vi "UHR-Fleezers Control (host) -Leonardo 04-2018 V2.vi"(0 "Tab Control":T5(tab)=enum."Trap Control (RF)") -> ()   [LabVIEW 2013] (continued)
-109.41462449554598, -109.30248158488335, -108.70735295493108, -109.9174743694956, -109.94232543385962, -110.71725446170196, -110.0346196158573, -110.34814317845934, -110.6651078322521, -107.55409880424479, -108.71734776861287, -109.50902203986271, -110.40207542979611, -108.7847687630861, -111.10599488129682, -109.30824728923263, -108.20134064331717, -110.55959112431609, -107.77099734327174, -110.23862843385446, -108.48520797666865, -108.54205896654946, -107.79288769037599, -109.84022250170581, -108.02758364115576, -109.35132492327935, -108.87009749667932, -109.86905123364855, -109.19826752168308, -106.835240323691, -109.37910022114056, -110.80633973102931, -109.12703823829597, -111.07432699570984, -111.8064506085314, -110.09349947650527, -108.66467295777367, -108.75119108236053, -112.63983351316729, -110.90940743670113, -110.27973159222081, -109.57141664526549, -108.61645363771719, -109.31742355616147, -109.5839599160637, -110.01188998365383, -110.01923429741011, -108.94779759137936, -108.26169431000017, -109.24553201026085, -109.95709526422822, -110.68677343596859, -108.7678734483002, -110.47090469179284, -110.31604700116512, -110.10256600741997, -109.76634647265719, -110.8830805828562, -109.94609564072982, -109.20662382740542, -108.12492970530919, -110.5274435478767, -108.02351960398035, -110.6264936805739, -107.14559226383577, -109.13821777857531, -111.05324489472586, -110.15190797512811, -107.96366234783144, -110.03950681967147, -109.17476300510336, -110.41251816187909, -111.39219865477246, -111.32530426869943, -109.97369363558423, -108.98666403063845, -109.62049358645565, -109.58130494498671, -111.72738873188874, -110.39825891106616, -108.57430325757545, -111.28625510212446, -108.77421250595326, -109.75025415031793, -109.51948456745635, -108.82129398637998, -109.81362137198361, -107.86292494316123, -107.49318292857053, -109.66948564589373, -109.54288390056654, -107.99912445612077, -110.3497559614379, -108.00549349666127, -110.01361420523357, -108.4977916421456, -109.67078387286976, -109.85678367732866, -112.01237658746248, -108.4855625950998, -110.84880875737286, -110.9178674382154, -110.44187536727453, -108.75076921971127, -110.04946286646651, -109.99780941000827, -110.14242932305507, -109.56343773672316, -109.6278993388131, -108.77419573790174, -109.10543670530926, -109.7801848627463, -110.30733124104881, -113.13440550301436, -109.32709134514755, -109.74136656933283, -110.01525283266193, -109.43924662938396, -110.25325289253, -107.75460576671303, -110.60057027395933, -110.71458404922404, -110.15788509050662, -110.69167485018224, -110.96006652476157, -111.01156633983031, -111.6058448010008, -109.51364005052672, -109.76058205940885, -108.43421621088261, -109.47973949170208, -109.25533250208288, -109.47422603921065, -111.36411644613841, -107.27566171102698, -110.45098686173688, -109.93589296291184, -109.03803734663714, -110.53118128434016, -110.2408872254969, -110.0532234862915, -109.94185495614619, -110.2662004220774, -109.51094016962288, -108.5210104215432, -108.13691752270934, -110.18460088390265, -108.32609309150783, -109.89652230508281, -109.80923900768477, -109.01917388968883, -110.01248300968739, -109.43415605440147, -108.09823485138017, -107.40637725320931, -109.40632232658412, -111.97981999127656, -111.16609811629485, -111.64500793960192, -110.99793748693381, -109.55531276386903, -110.2535662621666, -108.17429802469516, -109.09425673355422, -110.23187110421917, -110.55358397926925, -109.93461124753053, -109.55604345832225, -109.44569510408274, -109.72185151080762, -109.52963702944834, -109.2303630328152, -109.74819502244243, -109.3932530349457, -109.17096788339686, -110.46153727064616, -113.1073731246639, -109.43753070459397, -108.13332547768168, -109.42294574929969, -108.45798401969856, -110.29453435046327, -112.66249403705643, -108.78314667434937, -105.9634478773668, -109.14327524669528, -108.50645190860273, -100.81571594994128, -104.4482859840643, -110.68926237051092, -109.12362553230196, -109.45234390564677, -107.91461416156068, -110.67788819353727, -110.05744935668449, -111.78333392154664, -106.83628914455993, -110.11115457346548, -109.13434608275826, -110.80006861194663, -110.35323502651462, -112.29149906501372, -109.01656376530778, -109.30871662948859, -109.79736315392456, -109.17848983603582, -108.09752397056482, -111.6039030763455, -109.27008844877828, -110.84475733314184, -109.72393917557073, -111.31060762894991, -110.78858793807466, -107.12841545099752, -109.54510865218204, -105.2805426080281, -106.28514149354733, -109.50656759582803, -110.14700878401054, -110.49737016725709, -109.19811547071924, -109.92527399676051, -110.7961615015146, -109.7447227818197, -109.49432012009893, -108.714081576733, -110.09766801550917, -109.08448507943001, -110.36154838733857, -109.86328656267403, -109.21144237434696, -112.4145136888034, -108.57567151011159, -109.66748589540896, -109.72985837578446, -109.29989238126763, -109.85868902806475, -111.01778182304162, -111.23625326328558, -110.01270868104203, -109.27067928081415, -109.71171312410247, -109.28697459293629, -110.67868067201007, -110.91353786857455, -111.21479955051575, -109.11315965407708, -109.40418681804496, -107.80511819596003, -107.37201025889816, -111.81969609169838, -109.89875624306032, -110.29328043898657, -109.74853280072202, -111.39527865400605, -109.47746221101964, -111.75141177452517, -109.31325306583483, -109.30117448911659, -109.3997781364162, -109.45356931295724, -109.60585285774386, -111.33951689512735, -107.74187210470228, -109.62706021606415, -108.72139655505221, -109.79552836110567, -110.64354037499807, -110.96138240913136, -110.02215059889615, -110.92978442698893, -110.0620778287114, -110.85019647293322, -111.77397403227091, -109.81257196800128, -109.15643451383403, -110.72777566469594, -108.7463769025616, -109.80959395914073, -111.24500986151126, -110.48863498350322, -110.30863780110901, -109.79331354195703, -110.34087081762074, -109.45183222569266, -109.6440990067103, -111.15034876658994, -112.14912485578341, -111.8886180186196, -110.57054820211916, -111.07556239924551, -110.5872832735073, -110.28912501038172, -108.91501133754849, -111.44575118962761, -109.90799859177967, -109.74421995550023, -108.70941446115883, -110.28822893097275, -109.70039554000401, -110.33701797570251, -110.79445894683306, -109.57694314608153, -108.816904416038, -109.66517126767175, -109.39501469321644, -110.85775022889956, -109.3689402795614, -112.09107318723095, -110.67985626248422, -110.32971146814747, -112.08166943494875, -109.93955548712543, -109.31722953035252, -110.2062913031861, -108.22565380081006, -110.680898028151, -111.95386604441454, -110.83354130587097, -108.5873626748948, -111.97536144124408, -109.23944159551515, -111.57859477689586, -110.80135186615524, -110.4800953731021, -110.14040729648133, -109.25873050390551, -108.87000960474569, -110.97091597211167, -110.15787270199012, -111.62434537618091, -108.5421625277294, -110.42258666403919, -110.96896115868603, -108.98253068925274, -109.54245055160168, -110.28051096122468, -109.48060498658319, -109.77618362117276, -111.64513838754992, -111.13945484239875, -110.18094280356001, -110.43757222770748, -110.81588360154201, -110.11656805555333, -108.47936291282355, -109.16476249859961, -109.3549985917136, -110.77753190334253, -111.46065694661178, -110.40387985996301, -109.95673803226478, -111.58660981285446, -108.59894875229345, -109.37333363882607, -110.26849699991793, -109.30500469266264, -109.23789020998296, -110.82000706486865, -109.25927538839868, -111.03285659417519, -111.08899832832414, -110.69361682858042, -109.45187168573815, -109.9614018482838, -109.70209527974106, -112.11903952100165, -109.59713611623246, -110.70292028698111, -110.12743849746808, -110.63315585514292, -108.60450276298175, -109.32832664986026, -109.99753023477764, -109.46644696130294, -109.1781290160558, -111.58830180575129, -111.67229040267557, -111.3750024136205, -108.33616679452298, -109.99797067800029, -110.50892429124391, -108.66074740829372, -111.17094662568759, -109.87538933985836, -109.152526628291, -110.44623159817101, -110.21603106403009, -110.64376935639365, -109.36897426842583, -108.67303022227141, -109.89327693080823, -111.50442955563923, -111.37532237834381, -109.38132821290205, -109.73509680539144, -110.53918379735906, -111.22869870340647, -109.39977573957616, -110.3674665334106, -110.5366125953241, -109.99025356764304, -109.97300035646616, -109.87631077033762, -109.64608829594286, -113.02486102973394, -108.26250283140733, -109.62234918138763, -111.18766216512655, -110.33666026406992, -110.5808115327039, -108.2971671321189, -110.10964334161903, -110.61254021379767, -109.89852549557533, -110.16562049054073, -109.41433790018287, -111.2453823439446, -110.45554802599901, -113.11454453784393, -110.7333866145056, -110.00858191882439, -108.54745315874294, -110.08430415376903, -111.9006972727596, -110.3031506154679, -110.26331790366497, -109.36797925566673, -109.04860552478912, -111.83514212681175, -111.38960737633833, -109.01429665187288, -110.96404839103826, -108.95488871107163, -109.09652004914592, -111.884304581971, -110.57566691021339, -111.95113404442795, -110.13677174050159, -108.10078686353354, -107.69442565416006, -112.42676605669463, -109.12681161784135, -109.23120766087519, -110.57649395555585, -110.22143082743162, -108.40065951773644, -109.46923168308618, -111.39095086729745, -110.46375658526013, -111.45145283328486, -112.22610823637353, -110.61090190564383, -112.22250292674809, -111.7379343196361, -110.18530386733481, -108.93867365671692, -111.89304844956082, -109.06146134986984, -110.98405731832798, -109.76366821333497, -108.08326795663608, -109.95041147835065, -112.94140614324155, -111.79814935135965, -108.07337559063119, -109.13733403265212, -111.74906646037496, -111.12228668433455, -110.02899450462209, -110.22237716929811, -109.0224776891049, -110.18135850497721, -113.32516073881047, -111.3576490243877, -110.60510094465171, -109.6935518470342, -110.36313473154901, -111.95933240129618, -109.49625308071019, -109.18827910216122, -110.54311407822692, -108.4811035913567, -112.81280225723607, -108.86530665787413, -110.85796435061886, -110.40059714639627, -108.19250716343407, -108.96956521802292, -108.61281798886506, -109.78061525370413, -111.58885511891798, -109.06279169160345, -111.43043988466789, -111.63169336321079, -109.54702536206447, -109.62860636296405, -109.47865811135546, -108.02265793654806, -109.97461304995515, -110.72549884050886, -111.57309413919933, -110.03317891949746, -110.39570411598524, -110.27606115470397, -110.63294457306095, -110.71821689302902, -110.38076268941819, -111.51223508887897, -110.40703572670697, -112.24933273737743, -109.74954300082398, -108.46020292937696, -111.05315219575881, -110.38635148390118, -109.58268303790976, -112.34211536832117, -108.45894118755307, -108.96463982695337, -110.56040438523046, -110.67803313671729, -111.07349872375121, -110.42184162876096, -111.82081126435692, -108.85923651136297, -112.57723799596502, -113.65690874668172, -112.62314325834605, -110.70357529341362, -110.959925221544, -111.26336183001875, -108.1350700630152, -107.94545932312926, -111.17610778209841, -110.20386728310686, -108.55646511121591, -109.8400922569145, -111.73466587035968, -110.47272877573613, -108.33011124048193, -107.93042857580332, -108.60928277989103, -109.25240966798974, -108.96403833602028, -106.94222615757475, -109.37086694261907, -106.72743097285155, -109.03160193412796, -107.3549903889451, -106.8543848510082, -107.83503929060929, -106.30745467433752, -108.36915807168845, -107.13065938379303, -107.84769200880969, -106.08004345082777, -108.15244601930225, -108.37254117816573, -106.57863034819223, -108.1283698227614, -108.19776505569902, -107.58283412238643, -108.17365133196301, -108.6794309781181, -107.91552140588759, -111.60122989270022, -107.04360635941174, -111.55535949001795, -109.39870426166594, -109.55937904851662, -111.81389508925734, -109.88957041098786, -110.84764586896561, -110.59130246272693, -111.15944135223884, -110.19496154041607, -111.51861903129362, -110.74798816525838, -111.37312965175558, -110.10842817220238, -110.73198099204856, -111.36708667993291, -110.30840247819665, -110.11744489669044, -110.55237850846444, -108.2073528237766, -112.70750856801911, -110.99917956040802, -109.84949484779976, -111.3403161887679, -110.08924435263565, -110.17749213365616, -112.10849123224503, -110.94270741299202, -109.29350963424746, -110.33477486966507, -112.19620157705627, -111.45484078395934, -111.86858843505124, -110.22491147345858, -108.96177661263177, -108.67862820579893, -107.55155410582937, -108.27984439169573, -108.72682528077233, -110.64231212183269, -109.32873093119183, -112.98564364754564, -110.78933114228725, -108.50921025910479, -107.91087245586935, -112.57350030929283, -111.75871577457525, -108.42095298945462, -112.31266064114303, -110.1295657579673, -109.67444664474456, -110.33749884929306, -109.16098218724147, -109.63554874360221, -109.15892392675141, -111.90580809179818, -108.81196712336858, -111.42223552606656, -109.90571484965518, -109.99739812086352, -111.64103850263211, -111.31463957090885, -110.61247447444549, -110.20960333715526, -110.1707327818923, -109.70412636554525, -110.97278093107532, -110.24386747740314, -109.81378546061525, -110.83784085086458, -109.77357954318757, -111.22663832948885, -111.14563050139252, -110.87152231402447, -110.34246044319893, -109.97174570657546, -110.23599592972218, -111.08206161770731, -110.0073315341242, -111.11748366902188, -112.04005964728601, -109.81290191679287, -109.68543639040858, -112.01143296194752, -110.13641850530031, -108.19348942447623, -109.7534468948808, -109.36697824644176, -97.56454580435337, -104.97829040517887, -108.1539132982256, -110.048991273122, -107.46172505860011, -110.49269280640675, -109.94209901400029, -109.38576869679022, -111.43699124347364, -110.89973083498887, -111.2994445418276, -109.25144782032437, -113.25676258473536, -110.82078737428088, -109.97779571182073, -113.36294799183014, -111.38584551238931, -112.17267897274873, -108.56430946159155, -112.06841286528645, -110.36822473102735, -109.54758527532016, -110.48190506674653, -110.03535695860182, -109.3951469796576, -112.41910682256774, -111.38124138857238, -109.37850389100952, -111.65544568836181, -111.55876881606889, -109.3029209617236, -109.20030046194076, -108.82610577621037, -110.53329453526098, -109.96090595542142, -109.67834229432077, -110.62303603007352, -109.8388817181171, -109.22430039793213, -108.92749786663613, -110.05794249283548, -109.58534943218437, -110.50493887507297, -109.96373022997366, -111.0645036323456, -111.28501675364454, -109.77386932343008, -108.8952247140968, -110.09242801628717, -112.90943444063141, -110.72299296247249, -109.39094335967056, -110.95165384057718, -109.59809519359453, -110.4978602309597, -109.67109981692639, -111.2489619905986, -110.0937750887109, -109.76771021128954, -108.32976315018955, -111.3058145792439, -111.09464974601362, -110.99797900696136, -109.174315000222, -109.630351559617, -110.26289147175856, -110.22688407202517, -109.96748050100612, -112.13247633583758, -110.59994952890855, -110.93023020153811, -109.22457750926695, -110.26162558926984, -110.09713110375579, -111.73858994918328, -109.78183160058515, -109.7603471824367, -110.96016892586911, -111.23309626937036, -109.83093663960678, -114.05354944347246, -111.58202863059464, -110.42281828744524, -110.9521484732059, -112.5120328206343, -111.614891937737, -109.84428787405484, -111.61119567831453, -110.43095563229411, -111.71833448430398, -110.01132196809407, -109.37558169247951, -109.14091380022785, -110.42663661754088, -110.3598013572826, -109.78207135281417, -109.94058843992468, -109.88210328447205, -108.6217811850147, -107.17834387173707, -110.6447226986756, -111.10704778101115, -111.24396771977769, -110.47849395539598, -110.75150631628034, -109.67662689396347, -109.23145032835053, -108.83780193265358, -109.43468321661163, -102.22521103859944, -106.90009867479111, -108.91580608784525, -109.58671397003187, -110.56692028436989, -108.75103142680105, -111.00795573084157, -110.75039085328763, -109.48222099288613, -111.8621134816908, -110.26507966786443, -108.885924716389, -109.30841399453053, -112.3188631425597, -111.05677697153163, -108.8268571902449, -109.63028152237679, -114.82339015806369, -107.03435216376964, -111.34847692589166, -109.61354114874855, -112.32687758049907, -109.59816404231358, -111.64248480241805, -111.84075757907273, -110.44017657636552, -110.15181635726277, -111.93813663582833, -109.11826378836209, -109.99779889778326, -109.927119030584, -109.4389650887841, -111.52448814187727, -111.38736268499642, -110.51920914917922, -108.64230614681055, -108.90307263595304, -110.57246891832371, -109.65575340646116, -109.80359672370373, -108.83368585528197, -111.09385004343437, -108.83430005497769, -112.37784208819113, -109.50005381621696, -109.67421750136593, -111.39664088797532, -109.70867599669316, -109.52498993629875, -111.12341349673187, -110.0484037026941, -109.55138667646308, -111.06614422098669, -109.4785941493091, -110.25724082617013, -110.93950616855716, -110.53487953881397, -111.45722057988401, -110.32393446412904, -110.34361936710438, -108.6610336097813, -109.53631603696368, -108.06930707969195, -107.68056561368934, -108.73860971027449, -108.87111384617579, -108.40433837098611, -110.55999576884835, -106.83832061167207, -108.28786975902513, -109.18482905697472, -107.81071696594883, -107.91047268802457, -108.79613111673706, -111.05361322310213, -109.97897453479862, -109.12920563729425, -111.20538391490288, -109.26286135293664, -111.31400407177502, -109.92167984752287, -110.70854322826071, -108.59406515713611, -109.69371333227458, -109.36664873267313, -110.35521729513704, -110.40667924006368, -112.0181844636846, -111.01529188207431, -110.59246505728431, -109.95068312717868, -110.75807466894047, -109.58596443762707, -111.12127793384956, -109.59041634463125, -111.56255571372793, -110.43405578864342, -108.39660324329928, -111.1420710307505, -113.64788483868595, -111.67645688353934, -111.36878760365944, -109.68523694561108, -110.11608766310304, -109.25670490330123, -110.73546181099229, -111.77855039399805, -107.9662794718261, -109.67483334602832, -109.891258579519, -110.24757768183042, -109.50202895993814, -110.07763831916637, -109.96891925839451, -110.97268925927641, -109.31698133827767, -112.27933593506792, -110.36206721075725, -109.47379463718867, -110.27836850941338, -110.63738280998388, -111.3611682777485, -110.72689155959884, -111.55480904927032, -111.16689658479412, -110.35555645743601, -111.56609319131051, -110.88279459952174, -114.73607246523177, -109.95813757295693, -107.64639932425493, -111.26486783320321, -112.03946356928121, -111.8915972448334, -110.35245920812773, -110.83155104803564, -110.67437747473863, -110.9959682920065, -110.7815352345103, -111.13722283763049, -112.54797265493127, -110.06894780898469, -111.65186554925783, -111.83545188116254, -110.65894756123697, -108.48458025065264, -112.43760714427981, -114.1368408201927, -110.40065777895025, -110.1066998945526, -108.60654239598591, -110.5716060205154, -110.74257357180736, -111.1136089342442, -111.53539811075092, -113.2559601458872, -109.2003227548348, -110.42285840441025, -111.4086884998834, -111.61503050693868, -110.8194303494779, -108.9701587059964, -112.58521089509063, -110.10873915265242, -112.43440038319561, -110.03468788439882, -111.57896603236308, -110.21939233582523, -109.03614470500777, -110.11738923539659, -109.55359574898291, -110.416473622654, -109.4626868574157, -111.17164025076731, -110.3579689035081, -109.04338716157822, -112.36157114517567, -109.32125615922843, -112.71105693789394, -110.11019129547768, -108.96439402555632, -111.107663418839, -111.48306369859839, -110.9317530461794, -107.98628540532181, -111.1636972328743, -110.47837837583148, -109.04649309175733, -110.27110334963734, -111.35803630614352, -110.77259078859605, -111.46352820533895, -111.16789261049541, -109.2376344776325, -111.6795794983659, -111.74292205167644, -109.40835022991612, -111.02163652600731, -108.79482078001607, -110.6718658416566, -111.08747067599332, -112.15383726791498, -109.47049126158717, -109.061574046483, -111.23993049318979, -111.02521156588335, -109.46012868444186, -110.13918914826291, -112.08180381836377, -110.61929875223015, -111.4424805369965, -111.43420275069585, -109.71347556238717, -110.24726273025648, -109.7860268673935, -109.94126895018422, -111.41948668868926, -108.90555991781676, -110.81242861886172, -109.65007052722677, -112.12672329335953, -110.01123170946096, -111.13980448279096, -113.92013682657084, -108.6000853867411, -110.66793592761913, -110.61237681642844, -110.00839105230496, -109.38083187034974, -109.46119372195675, -110.3708067287448, -108.55518656223285, -113.33935987443276, -111.92184778392033, -111.80820718236087, -107.36852757311246, -109.51077803361602, -110.066791721019, -108.756710558672, -107.91391289865918, -110.72851430959301, -111.39074956442978, -112.928843679455, -109.87348280521556, -112.21371750380071, -110.82495902297394, -109.94006136010094, -110.58757785050143, -110.2790091349881, -111.43884888223081, -108.09540986530712, -109.63783244641691, -110.19577975613292, -110.01690033746098, -112.75938920157155, -109.27158857362184, -111.19519821680541, -110.14381902425255, -110.45955291199236, -111.55660330002316, -110.75604254261134, -111.02122553784838, -111.6490091060193, -110.93362819419399, -110.49033159684308, -110.70789549836027, -110.41991882034145, -110.0264093421208, -109.18432746063652, -110.15292268755287, -112.40733942236504, -111.32869665965416, -110.95418667871114, -111.14291568823575, -111.75555369152653, -112.98146297069803, -109.73870744292117, -111.33806139459435, -110.18838799491355, -112.60408243005732, -110.26112648646833, -110.58257045107274, -109.75155437454112]}, ...(2 in all)]
  in  "FFT 1 Choice 1":u16(ring) items=["T1 Y", "T1 X", "T1 Sum", "T2 Y", "T2 X", "T2 Sum", "T1 FB X", "T1 FB Sum", "T2 FB X", "T2 FB Sum", "PSD Y", "PSD X", "PSD Y Sum", "none"]
  in  "FFT 2 Choice 1":u16(ring)=3 items=["T1 Y", "T1 X", "T1 Sum", "T2 Y", "T2 X", "T2 Sum", "T1 FB X", "T1 FB Sum", "T2 FB X", "T2 FB Sum", "PSD Y", "PSD X", "PSD Y Sum", "none"]
  in  "FFT 1 Choice 2":u16(ring)=1 items=["T1 Y", "T1 X", "T1 Sum", "T2 Y", "T2 X", "T2 Sum", "T1 FB X", "T1 FB Sum", "T2 FB X", "T2 FB Sum", "PSD Y", "PSD X", "PSD Y Sum", "none"]
  in  "FFT 2 Choice 2":u16(ring)=4 items=["T1 Y", "T1 X", "T1 Sum", "T2 Y", "T2 X", "T2 Sum", "T1 FB X", "T1 FB Sum", "T2 FB X", "T2 FB Sum", "PSD Y", "PSD X", "PSD Y Sum", "none"]
  in  "Compute FFT":bool
  in  "Reset FFT":bool
  in  "# Spectra to Ave.":dbl=25.0
  out "Ave. Time (s)":dbl=1.5
  out "1 Channel":waveform(dbl)(graph)={"t0"=timestamp(0 s since 1904-01-01), "dt"=1.4999999999999999e-05, "Y"=array[20000 elements], "attributes"=variant("NI_ChannelName"=variant(string "T1 Y"))}
  out "Slow mean":dbl=-0.021350993491001932 format="%0.2f"
  in  "Slow mean N ave.":dbl=1.0 min=1.0 step=1.0
  out "Mean Intensity":dbl=-0.021350993491001957
  out "Sigma":dbl=0.006231607115497778
  out "Sigma/Mean":dbl=-0.2918649719098079
  in  "Subtract mean":bool
  in  "High Res. Display":u16(ring) items=["T1 Y", "T1 X", "T1 Sum", "T2 Y", "T2 X", "T2 Sum", "T1 FB X", "T1 FB Sum", "T2 FB X", "T2 FB Sum", "PSD Y", "PSD X", "PSD Y Sum"]
  out "APD 1 Rate (Hz)":dbl format="%#_3p"
  out "Feedback overload":bool
  in  "T2 for asymmetric\n(MHz)":dbl=85.0
  in  "Middle freq for \nsymmetric (MHz)":dbl=78.0
  in  "Symmetric manual \ntrap motion":bool
  out "Stage Moving":bool
  in  "Read Cal":bool
  in  "Confocal Linescan":bool
  in  "Speed (nm/s)":dbl=100.0
  in  "Furthest Withdraw (MHz)":dbl=15.0
  in  "Confocal Image":bool
  in  "Round T1 X":bool caption="Round"
  in  "T1 offset_x (mV)":dbl=44.132512662199076 format="%#_2g"
  in  "T1 kappa_x (pN/nm)":dbl=0.1608167093260824 min=0.0 step=0.001 format="%#_2g"
  out "Time (s)":dbl=40.5
  out "Total Time (s)":dbl=60.0
  in  "Start Saving":bool
  in  "Cal sets to save":u32=50 min=1 step=1
  in  "Comment (data description)":string="testing confocal setup"
  out "Calibrating Trap...":bool
  in  "Trap 2 (ON/OFF)":bool=TRUE
  in  "Trap 1 (ON/OFF)":bool=TRUE
  in  "Save Calibration":bool
  in  "N sets to save":u32=200 caption="N Sets"
  in  "Save N Sets":bool
  out "Save file name":path=path "I:/Data/160525/160525_043.dat"
  in  "Save ave N":dbl=500.0 caption="Averaging Factor"
  out "Saving...":bool
  in  "Stop Saving":bool
  out "Progress":u16(slide) scale=0.0..100.0
  out "Manipulating Trap":bool
  out "Buffer Status":dbl(slide) scale=0.0..1.0
  out "Overflow (data lost)":bool
  in  "Reset":bool
  out "Data Rate (Hz)":dbl=66666.66666666667 caption="Trap Data Rate (Hz)" format="%#_3p"
  out "Data Period (s)":dbl=1.4999999999999999e-05 caption="Trap Data Period (s)" format="%#_6p"
  out "Save Data Rate (Hz)":dbl=133.33333333333334 caption="Rate (Hz)" format="%#_6p"
  out "Save Data Period (s)":dbl=0.0075 caption="Period (s)" format="%#_6p"
  in  "T1 alpha_x (nm/V)":dbl=701.8425766517444 step=10.0 format="%#_3g"
  in  "T2 alpha_x (nm/V)":dbl=806.869454518421 step=10.0 format="%#_3g"
  in  "T2 kappa_x (pN/nm)":dbl=0.13871102209446912 min=0.0 step=0.001 format="%#_2g"
  in  "T2 offset_x (mV)":dbl=-16.403354316809207 format="%#_2g"
  in  "BD 1 Frequency 2 (MHz)":dbl=90.0 caption="T2 X (MHz)" min=60.0 max=90.0 step=1.0 format="%#_6p"
  in  "Green Laser ON/Interlacing":bool
  in  "Round T2 X":bool caption="Round"
  in  "AO1":dbl(slide) caption="Confocal Y (V)" min=0.0 max=10.0 step=0.01 scale=0.0..10.0 scale format="%_1f"
  in  "AO2":dbl(slide) caption="Confocal X (V)" min=0.0 max=10.0 step=0.01 scale=0.0..10.0 scale format="%_1f"
  in  "Trap Raster Scan":bool
  out "Raster Scanning...":bool
  in  "Trap Delta (MHz)":dbl=20.0 step=1.0
  in  "Trap Intensity\nSetpoints (V)":cluster{"Set 1":dbl, "Set 2":dbl}={"Set 1"=3.0921353801080356, "Set 2"=2.9123813592944123}
  in  "Index":dbl=43.0 caption="Save File Index" min=1.0 step=1.0
  in  "BD 1 Frequency 1 (MHz)":dbl=70.0 caption="T1 X (MHz)" min=60.0 max=90.0 step=1.0 format="%#_6p"
  in  "Goto Top (F6)":bool
  in  "Save":bool
  in  "Capture":bool
  out "?":cluster{"x":string, "y":string, "z":string}={"x"="N.D.\r\n", "y"="N.D.\r\n", "z"="N.D.\r\n"}
  in  "Capture Locations":i32(listbox)=2
  out "X Pos":string="-0.85624\r\n"
  out "Y Pos":string="0.27735\r\n"
  out "Z Pos Pos":string="0.05734\r\n"
  out "X Motion":string="1\r\n"
  out "Y Motion":string="1\r\n"
  out "Z motion":string="1\r\n"
  in  "Goto Bottom (F7)":bool
  in  "Goto Exp (F8)":bool
  in  "Main:":bool caption="Inject Pump 3"
  in  "Inject Top:":bool caption="Inject Pump 1"
  in  "Shunt:":bool
  in  "Inject Bottom":bool
  in  "Scan Range (nm)":dbl=1683.3000000000002
  out "Current Position":dbl[](array[numeric])=[4.2944, 4.91027471, 2.9278058] format="%7_7g"
  in  "Position Label 5":string="upper flow spot" caption="5"
  in  "Position 1 Label":string="Top capillary (SA beads)" caption="1"
  in  "Position 2 Label":string="Bottom capillary (AD) beads)" caption="2"
  in  "Position 3 Label":string="lower flow spot (ATP)" caption="3"
  in  "Position 4 Label":string="Dump beads" caption="4"
  out "Pump 3 cont disp":string="Left: ADig beads"
  out "Pump 1 cont disp":string="Right: DNA beads "
  in  "Ch 1 Inject Rate (ul/h)":dbl=50.0
  in  "Pump write delay (ms)":dbl=300.0
  in  "All Pump Parameters":T6={"Pump 1"={"Diameter (mm)"=4.61, "Units"=4.0, "Volume"=100.0, "Rate"=50.0}, "Pump 2"={"Diameter (mm)"=4.61, "Units"=3.0, "Volume"=0.0, "Rate"=0.0}, "Pump 3"={"Diameter (mm)"=4.61, "Units"=4.0, "Volume"=100.0, "Rate"=250.0}}
  in  "Ch 2 Inject Volume (uL)":dbl=100.0
  in  "Pump pause delay (ms)":u32
  in  "Ch 3 Inject Volume (uL)":dbl=100.0
  in  "Ch 3 Inject Rate (ul/h)":dbl=250.0
  in  "Flush Center Ch Volume (uL)":dbl=15.0
  in  "Flush Center Ch Rate (ul/m)":dbl=100.0
  in  "Inject Valve B":bool caption="Inject Pump 2\n(Flush Center)"
  in  "Total Volume\nFlushed (uL)":dbl
  in  "Tab Control 2":T7(tab)=enum."Feedback on Trap Position"
  in  "RF phase reset before cycles":bool
  in  "Phase increment trap 2":fxp<+/-,64,32>
  in  "Phase increment trap 1":fxp<+/-,64,32>
  in  "Phase offset method":u8=3
  in  "Next trap write delay (ticks)":u16
  out "FPGA error out":errorcluster
  out "Total Counts (ticks)":u32=600
  in  "Trap ON/OFF X or Y Amp?":bool=TRUE
  in  "Oscillate Set 2":bool
  in  "Trap 1 ON":bool=TRUE
  in  "Number Interlace Sets":u8=3 min=1 max=3
  in  "DIO count 3 (ticks)":u32=200
  in  "DIO count 2 (ticks)":u32=200
  in  "DIO count 1 (ticks)":u32=200
  in  "BD 2 Amplitude 3 (%)":dbl min=0.0 max=75.0 step=1.0
  in  "BD 2 Amplitude 2 (%)":dbl min=0.0 max=75.0 step=1.0
  in  "BD 2 Amplitude 1 (%)":dbl min=0.0 max=75.0 step=1.0
  in  "BD 1 Amplitude 3 (%)":dbl min=0.0 max=75.0 step=1.0
  in  "BD 1 Amplitude 2 (%)":dbl=42.0 min=0.0 max=75.0 step=1.0
  in  "BD 1 Amplitude 1 (%)":dbl=40.0 min=0.0 max=75.0 step=1.0
  in  "BD 2 Frequency 3 (MHz)":dbl=26.0 min=60.0 max=90.0 step=1.0 format="%#_6p"
  in  "BD 1 Frequency 3 (MHz)":dbl=70.0 min=60.0 max=90.0 step=1.0 format="%#_6p"
  in  "BD 2 Frequency 2 (MHz)":dbl=26.0 min=60.0 max=90.0 step=1.0 format="%#_6p"
  in  "BD 2 Frequency 1 (MHz)":dbl=26.0 min=60.0 max=90.0 step=1.0 format="%#_6p"
  in  "Not-Interlacing Set":enum32{"Set 1", "Set 2", "Set 3"}(radio)
  in  "Interlace":bool=TRUE
  in  "Trap 2 ON":bool=TRUE
  in  "Trap 3 ON":bool
  in  "Scan axis 2":bool=TRUE
  in  "Osc. freq. (Hz)":dbl=0.25
  in  "Osc. amp. (MHz)":dbl=2.0 format="%1_3g"
  out "Coords":T8
  in  "Manipulation Scaling":cluster{"Horizontal":dbl, "Vertical":dbl}={"Horizontal"=0.075, "Vertical"=0.01}
  in  "Freq or Amp switch first":bool=TRUE
  in  "Swap F1 and F2":bool
  in  "Freq switch delay":u16=9
  in  "Amp switch delay":u16=4
  in  "Period":i64=2
  in  "Raster to target force?":bool
  in  "Raster target force (pN)":dbl=10.0
  in  "MCL Step Increment (V_int)":dbl=3.0
  out "Time to Finish All (min)":dbl=0.666 format="%#_2p"
  in  "Scan Speed (nm/s)":dbl=100.0
  in  "Step Size (nm)":dbl=1.0
  in  "MCL/AOM Scale Tweak":dbl=1.0
  in  "MCL Step Position Ratio":dbl=0.5
  in  "Move MCL Also?":bool
  out "Final sep (nm)":dbl=1590.0
  out "Initial sep (nm)":dbl=360.0
  out "Save index":dbl=43.0
  out "Final delta (MHz)":dbl=30.0
  out "Initial delta (MHz)":dbl=20.0
  out "Final freq. (MHz)":dbl=60.0
  out "Initial freq. (MHz)":dbl=70.0
  in  "Saved AOD Raster Scan Parameter Sets":T9(array[cluster])=[{"Scan Range AOD (nm) 2"=500.0, "Step Size AOD (nm) 2"=1.0, "Scan Speed AOD (nm/s) 2"=100.0, "Number of scans (AOD) 2"=1, "Label"="offset curve"}, {"Scan Range AOD (nm) 2"=1000.0, "Step Size AOD (nm) 2"=1.0, "Scan Speed AOD (nm/s) 2"=100.0, "Number of scans (AOD) 2"=1, "Label"="hp raster check"}, {"Scan Range AOD (nm) 2"=6.8, "Step Size AOD (nm) 2"=0.34, "Scan Speed AOD (nm/s) 2"=0.34, "Number of scans (AOD) 2"=1, "Label"="3.4 kbp - 1 bp steps"}]
  in  "Load parameters":bool
  out "Scan Range (MHz)":dbl=-10.0
  in  "Restart DMA? (AOD)":bool=TRUE caption="Restart DMA?"
  out "Incr. int (AOD)":i64=-5670036101
  out "Time/Scan (s) (AOD)":dbl=19.98 format="%#_2p"
  out "Data points/scans":dbl=2664000.0
  out "Data points/scan (f/b)":dbl=2664000.0
  in  "Save scans":bool=TRUE
  out "AOD Scan I":u64=2 caption="Scan I"
  in  "Continuous AOD Scanning":bool caption="Continuous Scanning"
  in  "Abort AOD Scan":bool caption="Abort Scan"
  in  "Scan BD":bool=TRUE
  out "Cycles/step (AOD)":u64=666 format="%.3p"
  in  "Number of F/B Scans (AOD)":u16=1 min=1
  out "Scan steps (AOD)":u64=2000
  out "Scan Increment (MHz)":dbl=-0.0050025012506253125
  out "AOD Scanning":bool caption="Scanning"
  in  "Start AOD Scan":bool caption="Start Scan"
  out "N sets should be saved":dbl=133.2
  out "Progress 2":u16(slide) caption="Progress" scale=0.0..100.0
  in  "Abort save 2":bool caption="Abort save"
  in  "Trap 1 Bead Size (nm)":dbl=2100.0
  in  "Trap 2 Bead Size (nm)":dbl=2100.0
  out "MCL Count":dbl=782931.6080202644
  out "Trap 2 amplitude":ext
  out "Trap 1 amplitude":ext
  in  "PID gains":T10={"proportional gain (Kc)"=0, "integral gain (Kc*Ts/Ti)"=5, "derivative gain (Kc*Td/Ts)"=0}
  in  "All FB On/Off":bool
  in  "AI2 to Setpoint":cluster{"Set 1":bool, "Set 2":bool}
  out "AI2 (V)":cluster{"Set 1":dbl, "Set 2":dbl}={"Set 1"=3.087557603686636, "Set 2"=2.914212469862972}
  in  "Reset Feedback":cluster{"Set 1":bool, "Set 2":bool}
  in  "Feedback On/Off":cluster{"Set 1":bool, "Set 2":bool}={"Set 1"=TRUE, "Set 2"=TRUE}
  in  "Semi Passive ON":bool
  in  "DNA stiffness (pN / nm)":dbl=0.1
  in  "Semi Passive mode":enum16{"None", "Use Feedback", "Sharp Jump"}(ring)
  in  "Jump Force (pN)":dbl
  in  "Auto read offset\ncorrection":bool=TRUE
  in  "Negate Diff?":bool
  in  "Diff. FB.":bool=TRUE
  in  "Dynamic Force FB":bool=TRUE
  in  "Reset Trap Pos. FB":bool
  in  "Tab Control 8":enum32{"Main Setting", "Details"}(tab)
  in  "Real time offset \ncorrection for setpoint":bool=TRUE
  in  "Setpoint correction\noffset file":path
  in  "Negate offset difference":bool
  out "B factor":dbl=0.9916156324677038
  in  "Trap Pos FB Int Count":u16=100
  in  "Trap Pos. FB Gains":T11={"proportional gain (Kc)"=20.0, "integral gain (Kc*Ts/Ti)"=3.0, "derivative gain (Kc*Td/Ts)"=0.0} {"proportional gain (Kc)" format="%.11g"; "integral gain (Kc*Ts/Ti)" format="%.11g"; "derivative gain (Kc*Td/Ts)" format="%.11g"}
  out "Offset file step size":dbl=0.1
  in  "Read setpoint correction\nfile":bool
  in  "Trap Pos. FB Offset Factor":i64
  in  "Trap Pos FB Negate Action":bool=TRUE
  in  "Trap Pos. FB Mult Factor":i64=8388608
  in  "Trap Pos. AI1 X Pre-scale":u16
  in  "Trap Pos. FB Range":T12={"output high"=0.999969482421875, "output low"=-1.0}
  out "Trap Pos FB Int Signal":fxp<+/-,24,9>=42.09515380859375 format="%.18g"
  out "Trap Pos FB Int-Norm Signal":fxp<+/-,16,1>=0.042083740234375 format="%.16g"
  in  "Set SP Using...":bool
  in  "Trap Pos FB Monitor\nT1 or T2":bool
  out "Trap X AI1 (DMA)":T13={"Set 1"=0.030731201171875, "Set 2"=-0.0113525390625}
  in  "N El. to Ave.":dbl=10000.0
  out "Trap Pos FB Action":i64=-32767
  out "Mean T1 Position (nm)":dbl=-4.784226348419907e-12 caption="Mean T1 (nm)" format="%0.2f"
  out "Trap 1 Position RMS (A)":dbl caption="RMS (Ang)"
  in  "Offset Values":T14={"Trap 1X offset"=array[500 elements], "Trap 2X offset"=array[500 elements]}
  in  "Setpoint offset\nCorrection values":dbl[](array[numeric])=[0.024496601698410773, 0.024671186719617436, 0.024845771740824106, 0.025020356762030765, 0.02519494178323743, 0.025369526804444095, 0.025544111825650764, 0.025718696846857424, 0.025893281868064093, 0.026067866889270756, 0.026242451910477423, 0.026417036931684082, 0.02659162195289075, 0.026766206974097418, 0.02694079199530408, 0.027115377016510744, 0.027289962037717407, 0.027464547058924076, 0.02763913208013074, 0.027813717101337402, 0.027988302122544065, 0.02816288714375073, 0.028337472164957394, 0.02851205718616406, 0.028686642207370723, 0.028861227228577393, 0.02903581224978405, 0.029210397270990722, 0.029384982292197385, 0.02955956731340405, 0.02973415233461071, 0.029908737355817377, 0.030083322377024047, 0.03025790739823071, 0.030432492419437372, 0.030607077440644035, 0.0307816624618507, 0.030956247483057368, 0.03113083250426403, 0.0313054175254707, 0.03148000254667736, 0.03165458756788402, 0.03182917258909068, 0.03200375761029735, 0.032178342631504014, 0.03235292765271068, 0.03252751267391735, 0.03270209769512401, 0.03287668271633068, 0.033051267737537346, 0.033225852758744005, 0.03340043777995067, 0.03357502280115733, 0.033749607822364, 0.033924192843570664, 0.03409877786477733, 0.034273362885983996, 0.034447947907190656, 0.03462253292839732, 0.03479711794960398, 0.03497170297081065, 0.035146287992017314, 0.03532087301322398, 0.035495458034430646, 0.035670043055637306, 0.03584462807684397, 0.036019213098050645, 0.036193798119257305, 0.03636838314046397, 0.03654296816167063, 0.0367175531828773, 0.03689213820408396, 0.03706672322529063, 0.037241308246497296, 0.037415893267703955, 0.03759047828891062, 0.03776506331011729, 0.03793964833132395, 0.03811423335253061, 0.03828881837373728, 0.038463403394943946, 0.038637988416150605, 0.03881257343735727, 0.03898715845856393, 0.0391617434797706, 0.03933632850097726, 0.03951091352218393, 0.039685498543390596, 0.03986008356459726, 0.04003466858580393, 0.040209253607010595, 0.040383838628217254, 0.04055842364942392, 0.04073300867063058, 0.040907593691837246, 0.04108217871304391, 0.04125676373425058, 0.041431348755457245, 0.0416059337766639, 0.041780518797870564, 0.04195510381907723, 0.042129688840283896, 0.04230427386149057, 0.04247885888269723, 0.042653443903903895, 0.04282802892511056, 0.04300261394631722, 0.04317719896752389, 0.043351783988730554, 0.04352636900993721, 0.04370095403114388, 0.043875539052350546, 0.04405012407355721, 0.04422470909476388, 0.04439929411597054, 0.044573879137177204, 0.04474846415838387, 0.044923049179590537, 0.045097634200797196, 0.04527221922200386, 0.04544680424321053, 0.045621389264417195, 0.04579597428562386, 0.04597055930683052, 0.04614514432803718, 0.046319729349243846, 0.04649431437045051, 0.04666889939165718, 0.046843484412863845, 0.04701806943407051, 0.04719256456184452, 0.04736536676840916, 0.04753446267808822, 0.047696991448649737, 0.04784953848765512, 0.04799284096907562, 0.048127712917801824, 0.048257934523222495, 0.04838705366421733, 0.04851995197559876, 0.04865949840047511, 0.04880178465045004, 0.0489357994772595, 0.04905304538798107, 0.0491519464532862, 0.049234486275402736, 0.04930263064515607, 0.04935733149089569, 0.04939552771001872, 0.04941451823245213, 0.04941830757306315, 0.049410747020732684, 0.049392795273013504, 0.049367258833286985, 0.049339629147657244, 0.049311849604908836, 0.04928407006216041, 0.049256290519411994, 0.04922851097666357, 0.04920073143391515, 0.04917295189116673, 0.04914517234841831, 0.049117392805669895, 0.049089613262921473, 0.04906183372017306, 0.04903405417742463, 0.04900627463467622, 0.0489784950919278, 0.048950715549179374, 0.04892293600643097, 0.04889515646368254, 0.048867376920934125, 0.0488395973781857, 0.04881181783543728, 0.04878403829268886, 0.04875625874994044, 0.048728479207192026, 0.0487006996644436, 0.04867292012169519, 0.04864514057894676, 0.04861736103619835, 0.048589581493449926, 0.048561801950701505, 0.04853402240795309, 0.04850624286520466, 0.04847846332245625, 0.04845068377970783, 0.04842290423695941, 0.048395124694210985, 0.04836734515146257, 0.04833956560871415, 0.04831178606596573, 0.048284006523217314, 0.048256226980468886, 0.04822844743772048, 0.04820066789497206, 0.048172888352223636, 0.048145108809475215, 0.048117329266726794, 0.04808954972397837, 0.04806177018122996, 0.048033990638481544, 0.048006211095733116, 0.0479784315529847, 0.04795065201023628, 0.04792287246748786, 0.04789509292473944, 0.04786731338199102, 0.0478395338392426, 0.04781175429649418, 0.04778397475374576, 0.047756195210997346, 0.047728415668248925, 0.047700636125500503, 0.04767285658275208, 0.04764507704000366, 0.04761729749725524, 0.047589517954506826, 0.047561738411758404, 0.04753395886900998, 0.04750617932626157, 0.04747839978351315, 0.047450620240764727, 0.047422840698016305, 0.047395061155267884, 0.04736728161251948, 0.047339502069771056, 0.047311722527022634, 0.04728394298427421, 0.04725616344152579, 0.04722838389877737, 0.047200604356028956, 0.047172824813280535, 0.047145045270532114, 0.0471172657277837, 0.04708948618503528, 0.04706170664228686, 0.047033927099538436, 0.047006147556790015, 0.0469783680140416, 0.04695058847129318, 0.04692280892854476, 0.046895029385796344, 0.04686724984304792, 0.0468394703002995, 0.04681169075755108, 0.04678391121480266, 0.04675613167205424, 0.046728352129305824, 0.0467005725865574, 0.04667279304380899, 0.04664501350106057, 0.046617233958312146, 0.046589454415563725, 0.046561674872815303, 0.04653389533006689, 0.046506115787318475, 0.046478336244570054, 0.04645055670182163, 0.04642277715907321, 0.04639499761632479, 0.04636721807357637, 0.046339438530827955, 0.04631165898807953, 0.04628387944533112, 0.0462560999025827, 0.04622832035983428, 0.046200540817085856, 0.046172761274337434, 0.04614498173158901, 0.04611720218884059, 0.04608942264609218, 0.046061643103343757, 0.04603386356059534, 0.04600608401784692, 0.0459783044750985, 0.04595052493235008, 0.04592274538960166, 0.045894965846853236, 0.045867186304104815, 0.0458394067613564, 0.045811627218607986, 0.045783847675859565, 0.045756068133111144, 0.04572828859036272, 0.0457005090476143, 0.04567272950486588, 0.04564494996211747, 0.04561717041936905, 0.04558939087662063, 0.04556161133387221, 0.04553383179112379, 0.04550605224837537, 0.045478272705626946, 0.045450493162878525, 0.04542271362013011, 0.045394934077381696, 0.045367154534633275, 0.045339374991884854, 0.04531159544913643, 0.04528381590638801, 0.04525603636363959, 0.04522825682089117, 0.045200477278142755, 0.045172697735394333, 0.04514491819264592, 0.0451171386498975, 0.04508935910714908, 0.045061579564400656, 0.045033800021652234, 0.04500602047890381, 0.04497824093615539, 0.044950461393406985, 0.04492268185065856, 0.04489490230791014, 0.04486712276516172, 0.0448393432224133, 0.04481156367966488, 0.044783784136916464, 0.04475600459416805, 0.04472822505141963, 0.04470044550867121, 0.044672665965922786, 0.044644886423174365, 0.044617106880425944, 0.04458932733767752, 0.04456154779492911, 0.044533768252180694, 0.04450598870943227, 0.04447820916668385, 0.04445042962393543, 0.04442265008118701, 0.04439487053843859, 0.04436709099569017, 0.04433931145294175, 0.04431153191019333, 0.04428375236744492, 0.044255972824696496, 0.044228193281948075, 0.044200413739199654, 0.04417263419645123, 0.04414485465370281, 0.0441170751109544, 0.04408929556820598, 0.04406151602545756, 0.04403373648270914, 0.04400595693996072, 0.0439781773972123, 0.043950397854463884, 0.04392261831171546, 0.04389483876896704, 0.04386705922621863, 0.043839279683470206, 0.043811500140721785, 0.04378372059797336, 0.04375594105522494, 0.04372816151247652, 0.04370038196972811, 0.04367260242697968, 0.043644822884231264, 0.04361704334148285, 0.04358926379873443, 0.04356148425598601, 0.043533704713237587, 0.043505925170489165, 0.04347814562774075, 0.04345036608499233, 0.043422586542243916, 0.043394806999495494, 0.04336702745674707, 0.04333924791399865, 0.04331146837125023, 0.043283688828501816, 0.0432559092857534, 0.04322812974300498, 0.04320035020025656, 0.04317257065750814, 0.04314479111475972, 0.043117011572011296, 0.04308923202926288, 0.04306145248651446, 0.04303367294376604, 0.043005893401017625, 0.0429781138582692, 0.04295033431552078, 0.04292255477277236, 0.04289477523002394, 0.04286699568727552, 0.0428392161445271, 0.042811436601778684, 0.04278365705903027, 0.04275587751628185, 
